vi "HT graph.vi"() -> ()   [LabVIEW 2023]
uses:
  <vilib>/Utility/file.llb/Read Delimited Spreadsheet (DBL).vi
panel:
  out "recovery":dbl
  out "stage5":dbl
  out "stage4":dbl
  out "stage3":dbl
  out "stage2":dbl
  out "stage1":dbl
  out "baseline":dbl
  out "Waveform Graph":dbl[](graph)
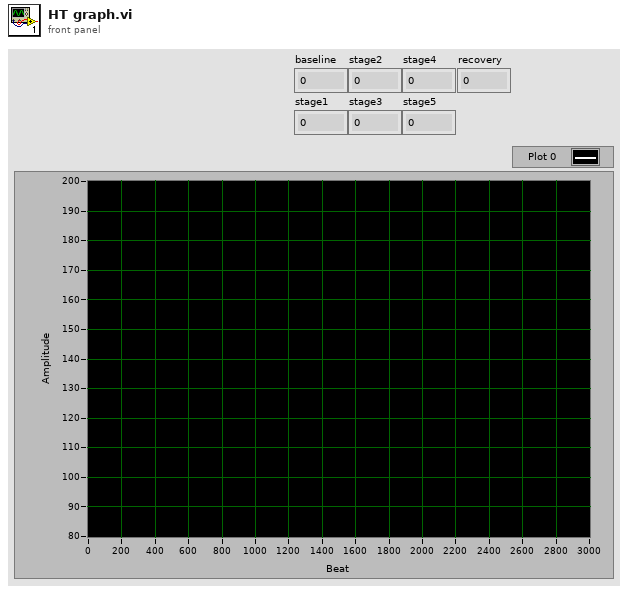
[diagram p1: front panel]
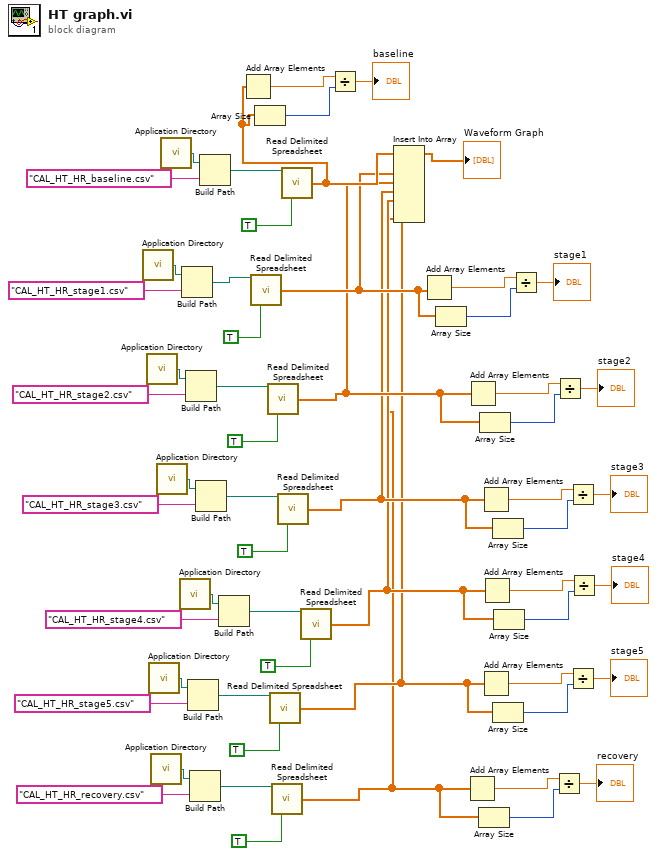
[diagram p0: block diagram]
diagram:
  n1 = call <vilib>:"Application Directory.vi"() -> ("Application Directory"=w53:path)
  n2 = call <vilib>:"Application Directory.vi"() -> ("Application Directory"=w49:path)
  n3 = call <vilib>:"Application Directory.vi"() -> ("Application Directory"=w37:path)
  n4 = call <vilib>:"Application Directory.vi"() -> ("Application Directory"=w32:path)
  n5 = call <vilib>:"Application Directory.vi"() -> ("Application Directory"=w45:path)
  n6 = call <vilib>:"Application Directory.vi"() -> ("Application Directory"=w57:path)
  n7 = call <vilib>:"Application Directory.vi"() -> ("Application Directory"=w41:path)
  n8 = Build Path(base path=w53, name or relative path="CAL_HT_HR_stage1.csv") -> (appended path=w50:path)
  n9 = Build Path(base path=w49, name or relative path="CAL_HT_HR_stage2.csv") -> (appended path=w46:path)
  n10 = Build Path(base path=w37, name or relative path="CAL_HT_HR_stage5.csv") -> (appended path=w34:path)
  n11 = Build Path(base path=w32, name or relative path="CAL_HT_HR_recovery.csv") -> (appended path=w29:path)
  n12 = Build Path(base path=w45, name or relative path="CAL_HT_HR_stage3.csv") -> (appended path=w42:path)
  n13 = Build Path(base path=w57, name or relative path="CAL_HT_HR_baseline.csv") -> (appended path=w54:path)
  n14 = Build Path(base path=w41, name or relative path="CAL_HT_HR_stage4.csv") -> (appended path=w38:path)
  n15 = call-poly <vilib>:"Read Delimited Spreadsheet.vi"("file path (dialog if empty)"=w50, "transpose? (F)"=TRUE) -> ("first row"=w21:dbl[])  [unwired: 8 in, 5 out]
  n16 = call-poly <vilib>:"Read Delimited Spreadsheet.vi"("file path (dialog if empty)"=w46, "transpose? (F)"=TRUE) -> ("first row"=w17:dbl[])  [unwired: 8 in, 5 out]
  n17 = call-poly <vilib>:"Read Delimited Spreadsheet.vi"("file path (dialog if empty)"=w34, "transpose? (F)"=TRUE) -> ("first row"=w5:dbl[])  [unwired: 8 in, 5 out]
  n18 = call-poly <vilib>:"Read Delimited Spreadsheet.vi"("file path (dialog if empty)"=w29, "transpose? (F)"=TRUE) -> ("first row"=w1:dbl[])  [unwired: 8 in, 5 out]
  n19 = call-poly <vilib>:"Read Delimited Spreadsheet.vi"("file path (dialog if empty)"=w42, "transpose? (F)"=TRUE) -> ("first row"=w13:dbl[])  [unwired: 8 in, 5 out]
  n20 = call-poly <vilib>:"Read Delimited Spreadsheet.vi"("file path (dialog if empty)"=w54, "transpose? (F)"=TRUE) -> ("first row"=w27:dbl[])  [unwired: 8 in, 5 out]
  n21 = Add Array Elements(numeric array=w27) -> (sum=w28:dbl)
  n22 = Array Size(array=w27) -> (size(s)=w26:i32)
  n23 = call-poly <vilib>:"Read Delimited Spreadsheet.vi"("file path (dialog if empty)"=w38, "transpose? (F)"=TRUE) -> ("first row"=w9:dbl[])  [unwired: 8 in, 5 out]
  n24 = Divide(x=w28, y=w26) -> (x/y=→"baseline":dbl)
  n25 = Insert Into Array(array=w27, new element #1=w21, new element #2=w17, new element #3=w13, new element #4=w9, new element #5=w5, new element #6=w1) -> (→"Waveform Graph":dbl[])  [unwired: 1 in]
  n26 = Add Array Elements(numeric array=w21) -> (sum=w24:dbl)
  n27 = Array Size(array=w21) -> (size(s)=w23:i32)
  n28 = Add Array Elements(numeric array=w1) -> (sum=w4:dbl)
  n29 = Add Array Elements(numeric array=w17) -> (sum=w20:dbl)
  n30 = Array Size(array=w1) -> (size(s)=w3:i32)
  n31 = Array Size(array=w17) -> (size(s)=w19:i32)
  n32 = Add Array Elements(numeric array=w13) -> (sum=w16:dbl)
  n33 = Add Array Elements(numeric array=w5) -> (sum=w8:dbl)
  n34 = Add Array Elements(numeric array=w9) -> (sum=w12:dbl)
  n35 = Array Size(array=w13) -> (size(s)=w15:i32)
  n36 = Array Size(array=w5) -> (size(s)=w7:i32)
  n37 = Array Size(array=w9) -> (size(s)=w11:i32)
  n38 = Divide(x=w24, y=w23) -> (x/y=→"stage1":dbl)
  n39 = Divide(x=w4, y=w3) -> (x/y=→"recovery":dbl)
  n40 = Divide(x=w20, y=w19) -> (x/y=→"stage2":dbl)
  n41 = Divide(x=w16, y=w15) -> (x/y=→"stage3":dbl)
  n42 = Divide(x=w8, y=w7) -> (x/y=→"stage5":dbl)
  n43 = Divide(x=w12, y=w11) -> (x/y=→"stage4":dbl)
